vi "Calculate loop iteration mean frequency.vi"(2 "Buffer length (10 points)":i32=10, 3 "Instant output during setup changes":bool) -> (0 "Refresh rate (Hz)":i32 format="Refresh Rate: %.0f Hz")   [LabVIEW 2017]
uses:
  <vilib>/Analysis/baseanly.llb/Mean (DBL).vi
  <vilib>/Analysis/NI_AALBase.lvlib
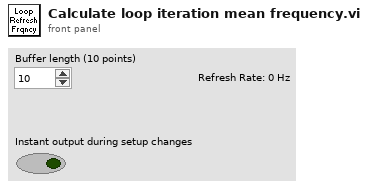
[diagram p1: front panel]
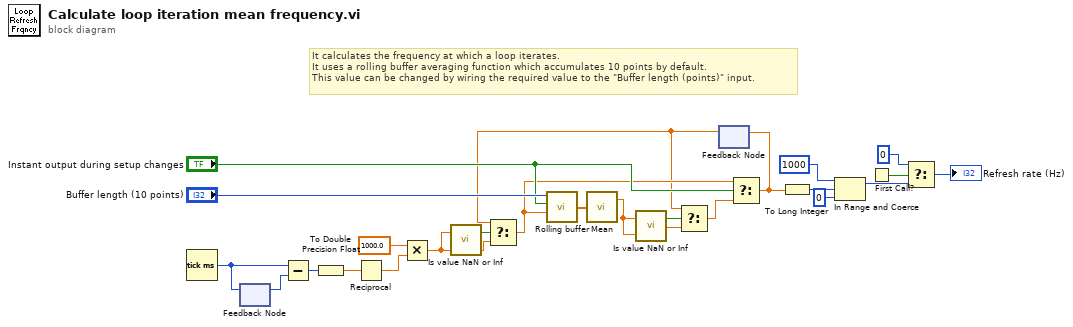
[diagram p0: block diagram]
diagram:
  # "It calculates the frequency at which a loop iterates.\nIt uses a rolling buffer averaging function which accumulates 10 points by default.\nThis value can be changed by wiring the required value to the \"Buffer length (points)\" input."
  n1 = Tick Count (ms)() -> (millisecond timer value=w22:u32)
  n2 = feedback-in #1(w22) -> ()
  n3 = feedback #1() -> (w21:u32)  [unwired: 1 in]
  n4 = Subtract(x=w22, y=w21) -> (x-y=w20:u32)
  n5 = To Double Precision Float(number=w20) -> (double precision float=w19:dbl)
  n6 = Reciprocal(x=w19) -> (1/x=w11:dbl)
  n7 = Multiply(x=1000.0, y=w11) -> (x*y=w4:dbl)
  n8 = call <userlib>:"Is value NaN or Inf.vi"("Value"=w4) -> ("NaN or Inf"=w3:bool)  [unwired: 2 in]
  n9 = feedback #2() -> (w6:dbl)  [unwired: 1 in]
  n10 = Select(t=w6, s=w3, f=w4) -> (s? t:f=w7:dbl)
  n11 = call "Rolling buffer.vi"("Value in"=w7, "Reset buffer"="Instant output during setup changes", "Buffer length (points)"="Buffer length (10 points)") -> ("Rolling buffer"=w8:dbl[])  [unwired: 8 in]
  n12 = call-poly <vilib>:"Mean.vi"("X"=w8) -> ("mean"=w2:dbl)  [unwired: 1 out]
  n13 = call <userlib>:"Is value NaN or Inf.vi"("Value"=w2) -> ("NaN or Inf"=w1:bool)  [unwired: 2 in]
  n14 = Select(t=w6, s=w1, f=w2) -> (s? t:f=w5:dbl)
  n15 = Select(t=w7, s="Instant output during setup changes", f=w5) -> (s? t:f=w9:dbl)
  n16 = feedback-in #2(w9) -> ()
  n17 = To Long Integer(number=w9) -> (32bit integer=w18:i32)
  n18 = In Range and Coerce(upper limit=1000, x=w18, lower limit=0) -> (coerced(x)=w13:i32)  [unwired: 1 out]
  n19 = First Call?() -> (First Call?: T/F=w15:bool)
  n20 = Select(t=0, s=w15, f=w13) -> (s? t:f=→"Refresh rate (Hz)":i32)
